vi "Divide By 1000 (1D).vi"(1 "X":dbl[](array[numeric])) -> (0 "X/1000":dbl[](array[numeric]))   [LabVIEW 2020]
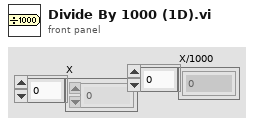
[diagram p1: front panel]
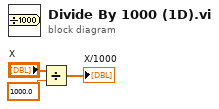
[diagram p0: block diagram]
diagram:
  n1 = Divide(x="X", y=1000.0) -> (x/y=→"X/1000":dbl[])
